vi "VCI Register Receive Callback.vi"(8 "error in (no error)":errorcluster, 10 "pReceiveCallBack":cluster{}, 11 "DevIndex":u32) -> (0 "error out":errorcluster, 3 "function return":u32)   [LabVIEW 2012, in "ControlCAN.lvlib"]
doc: "unsigned int WINAPI VCI_RegisterReceiveCallback(unsigned int DevIndex,PVCI_RECEIVE_CALLBACK pReceiveCallBack);"
uses:
  ControlCAN.lvlib
  Ginkgo_Driver.dll
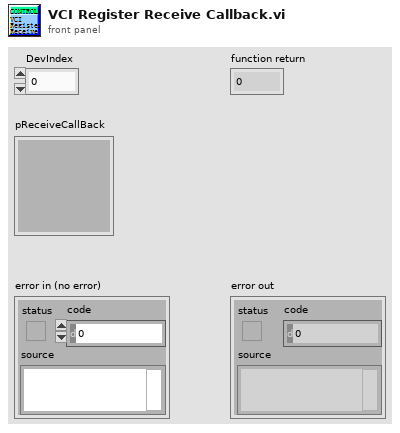
[diagram p1: front panel]
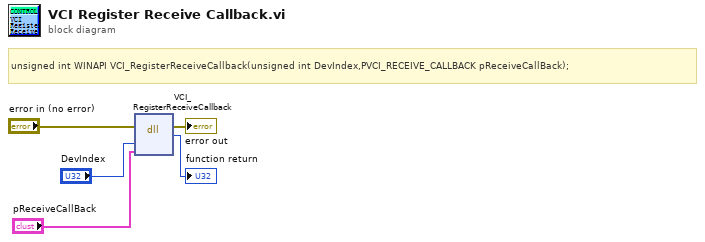
[diagram p0: block diagram]
diagram:
  # "unsigned int WINAPI VCI_RegisterReceiveCallback(unsigned int DevIndex,PVCI_RECEIVE_CALLBACK pReceiveCallBack);"
  n1 = dll-call lib="E:/Project/vt_ginkgo/truck/Ginkgo Driver/vs2010/Ginkgo_USB-I2C_API_v2.0.3.0/lib/labview_32bit/ControlCAN/Ginkgo_Driver.*" fn="VCI_RegisterReceiveCallback"(error in="error in (no error)", "DevIndex"="DevIndex", "pReceiveCallBack"="pReceiveCallBack") -> (error out=→"error out":errorcluster, →"function return":u32)  [unwired: 4 in, 1 out]
